vi "Lift.vi"() -> ()   [LabVIEW 2018]
uses:
  <vilib>/Rock Robotics/SystemInterfaces/DIO/FPGA_DIOChannel.ctl
  <vilib>/Rock Robotics/WPI/ThirdParty/Phoenix-LabVIEW/Motor Controller/Controls/CTRE_Phoenix_MotorControl_ControlMode.ctl
  Times/Times Global.vi
  Lift Global.vi
  <vilib>/addons/control/pid/pid.llb/PID (DBL).vi
  Robot Information/Robot Information Global.vi
  <vilib>/Rock Robotics/WPI/ThirdParty/Phoenix-LabVIEW/Motor Controller/Get/CTRE_Phoenix_MotorController_GetSelectedSensorData.vi
  Cargo Intake/Cargo Intake Global.vi
  <vilib>/addons/control/pid/NI_PID_pid.lvlib
panel:
  in  "Output Scalar":dbl=1.0 format="%#_13g"
  in  "t":dbl=0.65 format="%#_13g"
  in  "output range":cluster{"output high":dbl, "output low":dbl}={"output high"=0.95, "output low"=-0.8}
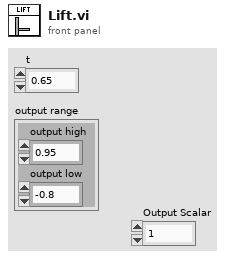
[diagram p1: front panel]
types:
  T1 = typedef "FPGA_DIOChannel.ctl" = enum8{"DIO 0", "DIO 1", "DIO 2", "DIO 3", "DIO 4", "DIO 5", "DIO 6", "DIO 7", "DIO 8", "DIO 9", "DIO MXP 0", "DIO MXP 1", "DIO MXP 2", "DIO MXP 3", "DIO MXP 4", "DIO MXP 5", "DIO MXP 6", "DIO MXP 7", "DIO MXP 8", "DIO MXP 9", "DIO MXP 10", "DIO MXP 11", "DIO MXP 12", "DIO MXP 13", "DIO MXP 14", "DIO MXP 15", "SPI Port CS1", "SPI Port CS2", "SPI Port CS3", "SPI Port MISO", "SPI Port MOSI", "Invalid"}
  T2 = typedef "WPI_MotorControlDeviceRef.ctl" = cluster{"DeviceStatus":errorcluster, "Type":T3, "PWM":cluster{"PWM Channel":T4, "DeadBand":T5}, "CAN":cluster{"Device Number":u8, "SetOutput VI Ref":variant, "GetOutput VI Ref":variant, "Enable VI Ref":variant, "Disable VI Ref":variant, "Data":variant}, "Invert":bool, "DIO PWM":cluster{"PWM \"Enable\" Channel":T4, "DIOChannel":T1, "PWM Rate":dbl}}
  T3 = typedef "WPI_MotorControlType.ctl" = enum16{"PWM", "CAN", "DIO PWM"}
  T4 = typedef "FPGA_DIOPWMChannel.ctl" = enum8{"PWM 0", "PWM 1", "PWM 2", "PWM 3", "PWM 4", "PWM 5", "PWM 6", "PWM 7", "PWM 8", "PWM 9", "PWM MXP 0", "PWM MXP 1", "PWM MXP 2", "PWM MXP 3", "PWM MXP 4", "PWM MXP 5", "PWM MXP 6", "PWM MXP 7", "PWM MXP 8", "PWM MXP 9", "Invalid"}
  T5 = typedef "WPI_PWMDeadband.ctl" = cluster{"Name":string, "maxPositivePwm":i32, "minPositivePwm":i32, "centerPwm":i32, "maxNegativePwm":i32, "minNegativePwm":i32, "angularRange":u16}
  T6 = typedef "WPI_DigitalInputDevRef.ctl" = cluster{"DevStatus":errorcluster, "DIO Channel":T1}
  T7 = typedef "CTRE_Phoenix_MotorControl_ControlMode.ctl" = u16
  T8 = cluster{"proportional gain (Kc)":dbl, "integral time(Ti, min)":dbl, "derivative time(Td, min) 2":dbl}
  T9 = enum16{"Hatch Panel Zone 1", "Hatch Panel Zone 2", "Hatch Panel Zone 3", "Cargo Zone 1", "Cargo Zone 2", "Cargo Zone 3", "Cargo Ship Zone"}
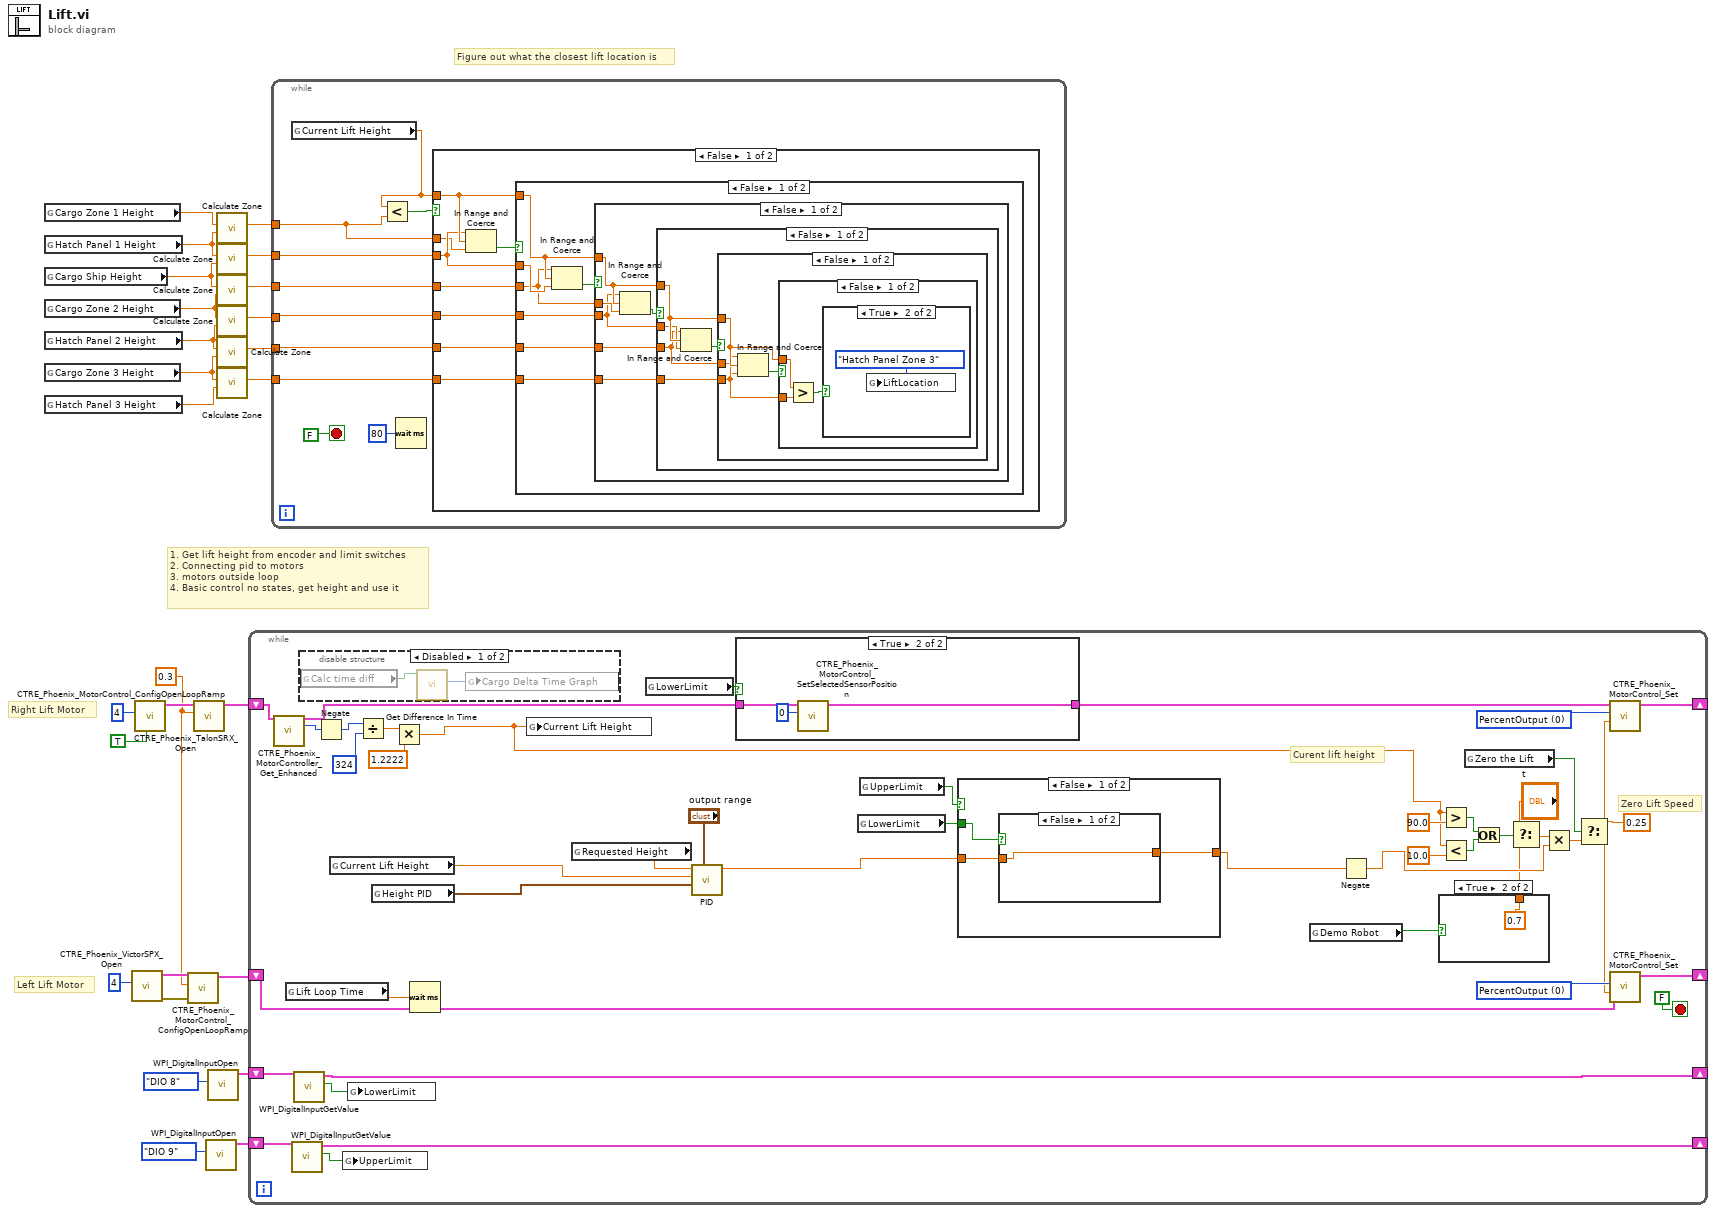
[diagram p0: block diagram]
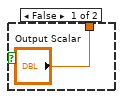
[diagram p2: hidden frame]
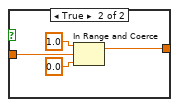
[diagram p3: hidden frame]
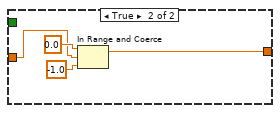
[diagram p4: hidden frame]
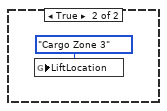
[diagram p8: hidden frame]
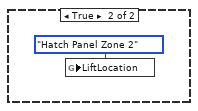
[diagram p9: hidden frame]
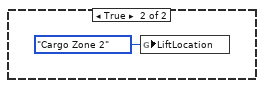
[diagram p10: hidden frame]
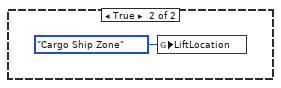
[diagram p11: hidden frame]
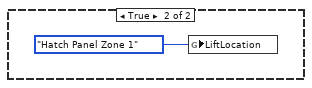
[diagram p12: hidden frame]
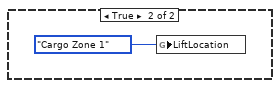
[diagram p13: hidden frame]
diagram:
  w2 = 0.3 ("secondsFromNeutralToFull")
  # "Left Lift Motor"
  # "Right Lift Motor"
  # "Figure out what the closest lift location is"
  # "1. Get lift height from encoder and limit switches\n2. Connecting pid to motors\n3. motors outside loop\n4. Basic control no states, get height and use it"
  n1 = global read "Lift Global.vi" "Cargo Zone 1 Height"() -> (w20:dbl)
  n2 = global read "Lift Global.vi" "Hatch Panel 1 Height"() -> (w26:dbl)
  n3 = global read "Lift Global.vi" "Cargo Ship Height"() -> (w25:dbl)
  n4 = global read "Lift Global.vi" "Cargo Zone 2 Height"() -> (w24:dbl)
  n5 = global read "Lift Global.vi" "Hatch Panel 2 Height"() -> (w23:dbl)
  n6 = global read "Lift Global.vi" "Cargo Zone 3 Height"() -> (w22:dbl)
  n7 = global read "Lift Global.vi" "Hatch Panel 3 Height"() -> (w21:dbl)
  n8 = call <vilib>:"CTRE_Phoenix_VictorSPX_Open.vi"("Device Number"=u8 4) -> ("error out"=w5:errorcluster, "CAN Talon SRX Ref"=w4:T2)  [unwired: 9 in]
  n9 = call <vilib>:"CTRE_Phoenix_TalonSRX_Open.vi"("Invert"=TRUE, "Device Number"=u8 4) -> ("CAN Talon SRX Ref"=w7:T2)  [unwired: 8 in, 1 out]
  n10 = call <vilib>:"CTRE_Phoenix_MotorControl_ConfigOpenLoopRamp.vi"("error in (no error)"=w5, "secondsFromNeutralToFull"=w2, "PhoenixMotorControlDevRef"=w4) -> ("PhoenixMotorControlDevRef"=w3:T2)  [unwired: 7 in, 1 out]
  n11 = call <vilib>:"CTRE_Phoenix_MotorControl_ConfigOpenLoopRamp.vi"("secondsFromNeutralToFull"=w2, "PhoenixMotorControlDevRef"=w7) -> ("PhoenixMotorControlDevRef"=w6:T2)  [unwired: 8 in, 1 out]
  n12 = call <vilib>:"WPI_DigitalInputOpen.vi"("DIO Channel"=FPGA_DIOChannel."DIO 9") -> ("DigitalInputDevRef"=w8:T6)  [unwired: 9 in, 1 out]
  n13 = call <vilib>:"WPI_DigitalInputOpen.vi"("DIO Channel"=FPGA_DIOChannel."DIO 8") -> ("DigitalInputDevRef"=w10:T6)  [unwired: 9 in, 1 out]
  n14 = call "Calculate Zone.vi"("Top Height"=w26, "Bottom Height"=w20) -> ("Midpoint"=w19:dbl)  [unwired: 9 in]
  n15 = call "Calculate Zone.vi"("Top Height"=w25, "Bottom Height"=w26) -> ("Midpoint"=w18:dbl)  [unwired: 9 in]
  n16 = call "Calculate Zone.vi"("Top Height"=w24, "Bottom Height"=w25) -> ("Midpoint"=w17:dbl)  [unwired: 9 in]
  n17 = call "Calculate Zone.vi"("Top Height"=w23, "Bottom Height"=w24) -> ("Midpoint"=w16:dbl)  [unwired: 9 in]
  n18 = call "Calculate Zone.vi"("Top Height"=w22, "Bottom Height"=w23) -> ("Midpoint"=w15:dbl)  [unwired: 9 in]
  n19 = call "Calculate Zone.vi"("Top Height"=w21, "Bottom Height"=w22) -> ("Midpoint"=w14:dbl)  [unwired: 9 in]
  n20 = while {
    shift-right: [w68] -> _
    shift-left: w6 -> [w61]
    shift-right: [w66] -> _
    shift-left: w3 -> [w65]
    shift-right: [w56] -> _
    shift-left: w10 -> [w57]
    shift-right: [w51] -> _
    shift-left: w8 -> [w52]
    stop <- FALSE stop-if-true
    w67 = T7 0 items=["PercentOutput"=0, "Position"=1, "Velocity"=2, "Current"=3, "Follower"=5, "MotionProfile"=6, "MotionMagic"=7, "MotionProfileArc"=10, "Disabled"=15] ("Control Mode")
    w69 = T7 0 items=["PercentOutput"=0, "Position"=1, "Velocity"=2, "Current"=3, "Follower"=5, "MotionProfile"=6, "MotionMagic"=7, "MotionProfileArc"=10, "Disabled"=15] ("Control Mode")
    # "Curent lift height"
    # "Zero Lift Speed"
    n21 = call-poly <vilib>:"CTRE_Phoenix_MotorController_Get_Enhanced.vi"("PhoenixMotorControlDevRef"=w61) -> ("PhoenixMotorControlDevRef"=w60:T2, "Position (Raw Sensor Units)"=w34:i32)  [unwired: 11 in, 2 out]
    n22 = global read "Times Global.vi" "Lift Loop Time"() -> (w71:dbl)
    n23 = call <vilib>:"WPI_DigitalInputGetValue.vi"("DigitalInputDevRef"=w52) -> ("Value"=w54:bool, "DigitalInputDevRef"=w51:T6)  [unwired: 8 in, 1 out]
    n24 = call <vilib>:"WPI_DigitalInputGetValue.vi"("DigitalInputDevRef"=w57) -> ("Value"=w55:bool, "DigitalInputDevRef"=w56:T6)  [unwired: 8 in, 1 out]
    n25 = disable-structure shown="Disabled" {
      frame Disabled {
        n26 = global read "Cargo Intake Global.vi" "Calc time diff"() -> (w91:bool)
        n27 = call "Get Difference In Time.vi"("Calculate Time Difference"=w91) -> ("Delta Time over Time"=w90:u32)  [unwired: 9 in, 1 out]
        n28 = global write "Times Global.vi" "Cargo Delta Time Graph"(w90) -> ()
      }
      frame Enabled {
      }
    }
    n29 = Negate(x=w34) -> (-x=w35:i32)
    n30 = global read "Lift Global.vi" "Current Lift Height"() -> (w62:dbl)
    n31 = global write "Lift Global.vi" "UpperLimit"(w54) -> ()
    n32 = global write "Lift Global.vi" "LowerLimit"(w55) -> ()
    n33 = Divide(x=w35, y=324) -> (x/y=w41:dbl)
    n34 = global read "Lift Global.vi" "Height PID"() -> (w63:T8)
    n35 = Multiply(x=w41, y=1.2222) -> (x*y=w28:dbl)
    n36 = Wait (ms)(milliseconds to wait=w71) -> ()  [unwired: 1 out]
    n37 = global write "Lift Global.vi" "Current Lift Height"(w28) -> ()
    n38 = global read "Lift Global.vi" "Requested Height"() -> (w29:dbl)
    n39 = global read "Lift Global.vi" "LowerLimit"() -> (w53:bool)
    n40 = call-poly <vilib>:"PID.vi"("output range"="output range", "PID gains"=w63, "process variable"=w62, "setpoint"=w29) -> ("output"=w31:dbl)  [unwired: 6 in, 1 out]
    n41 = case shown="True" w53 {
      tunnel: w60 -> [w86 w89]
      tunnel: [w86 w88] -> w59
      frame False {
      }
      frame True {
        n42 = call <vilib>:"CTRE_Phoenix_MotorControl_SetSelectedSensorPosition.vi"("New Sensor Position"=0, "PhoenixMotorControlDevRef"=w89) -> ("PhoenixMotorControlDevRef"=w88:T2)  [unwired: 8 in, 1 out]
      }
    }
    n43 = global read "Lift Global.vi" "LowerLimit"() -> (w33:bool)
    n44 = global read "Lift Global.vi" "UpperLimit"() -> (w32:bool)
    n45 = case shown="False" w32 {
      tunnel: w33 -> [w76 _]
      tunnel: [w75 w83] -> w30
      tunnel: w31 -> [w74 w82]
      frame False {
        n46 = case shown="False" w76 {
          tunnel: [w77 w81] -> w75
          tunnel: w74 -> [w77 w78]
          frame False {
          }
          frame True {
            n47 = In Range and Coerce(upper limit=1.0, x=w78, lower limit=0.0) -> (coerced(x)=w81:dbl)  [unwired: 1 out]
          }
        }
      }
      frame True {
        n48 = In Range and Coerce(upper limit=0.0, x=w82, lower limit=-1.0) -> (coerced(x)=w83:dbl)  [unwired: 1 out]
      }
    }
    n49 = global read "Robot Information Global.vi" "Demo Robot"() -> (w27:bool)
    n50 = Negate(x=w30) -> (-x=w44:dbl)
    n51 = case shown="True" w27 {
      tunnel: ["Output Scalar" 0.7 ("Output Scalar")] -> w43
      frame False {
      }
      frame True {
      }
    }
    n52 = Greater?(x=w28, y=90.0) -> (0:w47:bool)
    n53 = Less?(x=w28, y=10.0) -> (x < y?=w48:bool)
    n54 = global read "Lift Global.vi" "Zero the Lift"() -> (w38:bool)
    n55 = Or(x=w47, y=w48) -> (x .or. y?=w46:bool)
    n56 = Select(t="t", s=w46, f=w43) -> (s? t:f=w45:dbl)
    n57 = Multiply(x=w45, y=w44) -> (x*y=w39:dbl)
    n58 = Select(t=0.25, s=w38, f=w39) -> (s? t:f=w36:dbl)
    n59 = call <vilib>:"CTRE_Phoenix_MotorControl_Set.vi"("Output"=w36, "Control Mode"=w69, "PhoenixMotorControlDevRef"=w59) -> ("PhoenixMotorControlDevRef"=w68:T2)  [unwired: 7 in, 1 out]
    n60 = call <vilib>:"CTRE_Phoenix_MotorControl_Set.vi"("Output"=w36, "Control Mode"=w67, "PhoenixMotorControlDevRef"=w65) -> ("PhoenixMotorControlDevRef"=w66:T2)  [unwired: 7 in, 1 out]
  }
  n61 = while {
    tunnel: w19 -> [w97]
    tunnel: w18 -> [w96]
    tunnel: w17 -> [w95]
    tunnel: w16 -> [w94]
    tunnel: w15 -> [w93]
    tunnel: w14 -> [w92]
    stop <- FALSE stop-if-true
    n62 = global read "Lift Global.vi" "Current Lift Height"() -> (w98:dbl)
    n63 = Less?(x=w98, y=w97) -> (x < y?=w99:bool)
    n64 = Wait (ms)(milliseconds to wait=u32 80) -> ()  [unwired: 1 out]
    n65 = case shown="False" w99 {
      tunnel: w98 -> [w105 _]
      tunnel: w97 -> [w103 _]
      tunnel: w96 -> [w104 _]
      tunnel: w95 -> [w109 _]
      tunnel: w94 -> [w108 _]
      tunnel: w93 -> [w107 _]
      tunnel: w92 -> [w106 _]
      frame False {
        n66 = In Range and Coerce(upper limit=w104, x=w105, lower limit=w103) -> (In Range?=w102:bool)  [unwired: 1 out]
        n67 = case shown="False" w102 {
          tunnel: w105 -> [w112 _]
          tunnel: w104 -> [w111 _]
          tunnel: w109 -> [w110 _]
          tunnel: w108 -> [w116 _]
          tunnel: w107 -> [w115 _]
          tunnel: w106 -> [w114 _]
          frame False {
            n68 = In Range and Coerce(upper limit=w110, x=w112, lower limit=w111) -> (In Range?=w113:bool)  [unwired: 1 out]
            n69 = case shown="False" w113 {
              tunnel: w112 -> [w119 _]
              tunnel: w116 -> [w117 _]
              tunnel: w115 -> [w122 _]
              tunnel: w114 -> [w121 _]
              tunnel: w110 -> [w118 _]
              frame False {
                n70 = In Range and Coerce(upper limit=w117, x=w119, lower limit=w118) -> (In Range?=w120:bool)  [unwired: 1 out]
                n71 = case shown="False" w120 {
                  tunnel: w119 -> [w125 _]
                  tunnel: w122 -> [w123 _]
                  tunnel: w121 -> [w127 _]
                  tunnel: w117 -> [w124 _]
                  frame False {
                    n72 = In Range and Coerce(upper limit=w123, x=w125, lower limit=w124) -> (In Range?=w126:bool)  [unwired: 1 out]
                    n73 = case shown="False" w126 {
                      tunnel: w125 -> [w130 _]
                      tunnel: w127 -> [w129 _]
                      tunnel: w123 -> [w128 _]
                      frame False {
                        n74 = In Range and Coerce(upper limit=w129, x=w130, lower limit=w128) -> (In Range?=w131:bool)  [unwired: 1 out]
                        n75 = case shown="False" w131 {
                          tunnel: w130 -> [w134 _]
                          tunnel: w129 -> [w133 _]
                          frame False {
                            n76 = Greater?(x=w134, y=w133) -> (0:w132:bool)
                            n77 = case shown="True" w132 {
                              frame False {
                              }
                              frame True {
                                n78 = global write "Lift Global.vi" "LiftLocation"(T9."Hatch Panel Zone 3" ("LiftLocation")) -> ()
                              }
                            }
                          }
                          frame True {
                            n79 = global write "Lift Global.vi" "LiftLocation"(T9."Cargo Zone 3" ("LiftLocation")) -> ()
                          }
                        }
                      }
                      frame True {
                        n80 = global write "Lift Global.vi" "LiftLocation"(T9."Hatch Panel Zone 2" ("LiftLocation")) -> ()
                      }
                    }
                  }
                  frame True {
                    n81 = global write "Lift Global.vi" "LiftLocation"(T9."Cargo Zone 2" ("LiftLocation")) -> ()
                  }
                }
              }
              frame True {
                n82 = global write "Lift Global.vi" "LiftLocation"(T9."Cargo Ship Zone" ("LiftLocation")) -> ()
              }
            }
          }
          frame True {
            n83 = global write "Lift Global.vi" "LiftLocation"(T9."Hatch Panel Zone 1" ("LiftLocation")) -> ()
          }
        }
      }
      frame True {
        n84 = global write "Lift Global.vi" "LiftLocation"(T9."Cargo Zone 1" ("LiftLocation")) -> ()
      }
    }
  }
